vi "Error Checker.vi"(8 "error in (no error)":errorcluster, 11 "Initial States in":T1[](array[typedef])) -> (0 "error out":errorcluster, 3 "Initial States out":T1[](array[typedef]))   [LabVIEW 2017]
uses:
  Controls/HID State.ctl
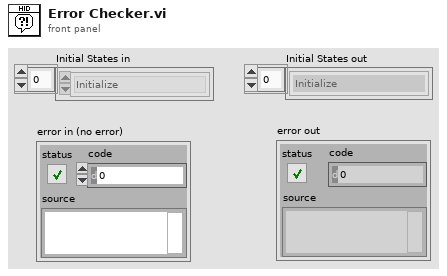
[diagram p1: front panel]
types:
  T1 = typedef "HID State.ctl" = enum16{"Initialize", "Set FPGA Parametes", "Set Camera Parameters", "Set LED Matrix Parameters", "Initialize FPGA Interface", "Initialize Camera", "Start FPGA VI", "Start Camera", "Wait for Event", "Update UI", "Acquire", "Process Image", "Get Boolean Arrays", "Send to FPGA", "Menu Pop-Up", "Menu Actions", "Handle Errors", "Close Camera", "Close FPGA", "Stop", "Exit"}
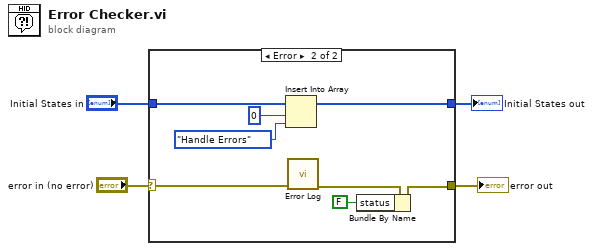
[diagram p0: block diagram]
diagram:
  n1 = case shown="Error" "error in (no error)" {
    selector: "error in (no error)" -> [w6 w10]
    tunnel: [w5 w14] -> w4
    tunnel: "Initial States in" -> [w5 w13]
    tunnel: [w6 w8] -> w1
    frame No Error {
    }
    frame Error {
      n2 = Insert Into Array(array=w13, index=0, new element=HID_State."Handle Errors" ("new element/subarray")) -> (w14:T1[])
      n3 = call "Error Log.vi"("error in (no error)"=w10) -> ("error out"=w9:errorcluster)  [unwired: 10 in]
      n4 = Bundle By Name(cluster=w9, "status"=FALSE) -> (w8:errorcluster)
    }
  }
  "Initial States out" <- w4
  "error out" <- w1
